vi "AllThingsBaxter_ROS_myRIO.vi"() -> ()   [LabVIEW 2015]
doc: "Collection of all ROS for LabVIEW VIs in the palette"
uses:
  ROS/MessageBuilding/std_msgs/subs/boolScalar.vi
  ROS/MessageBuilding/std_msgs/subs/durationScalar.vi
  ROS/MessageBuilding/std_msgs/subs/float32Scalar.vi
  ROS/MessageBuilding/std_msgs/subs/float64Scalar.vi
  ROS/MessageBuilding/std_msgs/subs/i8Scalar.vi
  ROS/MessageBuilding/std_msgs/subs/i16Scalar.vi
  ROS/MessageBuilding/std_msgs/subs/i32Scalar.vi
  ROS/MessageBuilding/std_msgs/subs/i64Scalar.vi
  ROS/MessageBuilding/std_msgs/subs/stringScalar.vi
  ROS/MessageBuilding/std_msgs/subs/timeScalar.vi
  ROS/MessageBuilding/std_msgs/subs/u8Scalar.vi
  ROS/MessageBuilding/std_msgs/subs/u16Scalar.vi
  ROS/MessageBuilding/std_msgs/subs/u32Scalar.vi
  ROS/MessageBuilding/std_msgs/subs/u64Scalar.vi
  ROS/Code/_ROSDefinition.vi
  ROS/MessageParsing/std_msgs/subs/parse_bool_scalar.vi
  ROS/MessageParsing/std_msgs/subs/parse_duration_scalar.vi
  ROS/MessageParsing/std_msgs/subs/parse_float32_scalar.vi
  ROS/MessageParsing/std_msgs/subs/parse_float64_scalar.vi
  ROS/MessageParsing/std_msgs/subs/parse_i16_scalar.vi
  ROS/MessageParsing/std_msgs/subs/parse_i32_scalar.vi
  ROS/MessageParsing/std_msgs/subs/parse_i64_scalar.vi
  ROS/MessageParsing/std_msgs/subs/parse_i8_scalar.vi
  ROS/MessageParsing/std_msgs/subs/parse_string_scalar.vi
  ROS/MessageParsing/std_msgs/subs/parse_time_scalar.vi
  ROS/MessageParsing/std_msgs/subs/parse_u16_scalar.vi
  ROS/MessageParsing/std_msgs/subs/parse_u32_scalar.vi
  ROS/MessageParsing/std_msgs/subs/parse_u64_scalar.vi
  ROS/MessageParsing/std_msgs/subs/parse_u8_scalar.vi
  ROS/MessageParsing/std_msgs/subs/parse_bool_array.vi
  BaxterVIs/LeftGripper.vi
  BaxterVIs/BothArmsPosition.vi
  BaxterVIs/read_green_level.vi
panel:
  out "ROS Master":string="192.168.1.110:11311"
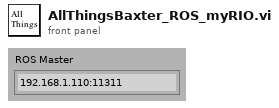
[diagram p1: front panel]
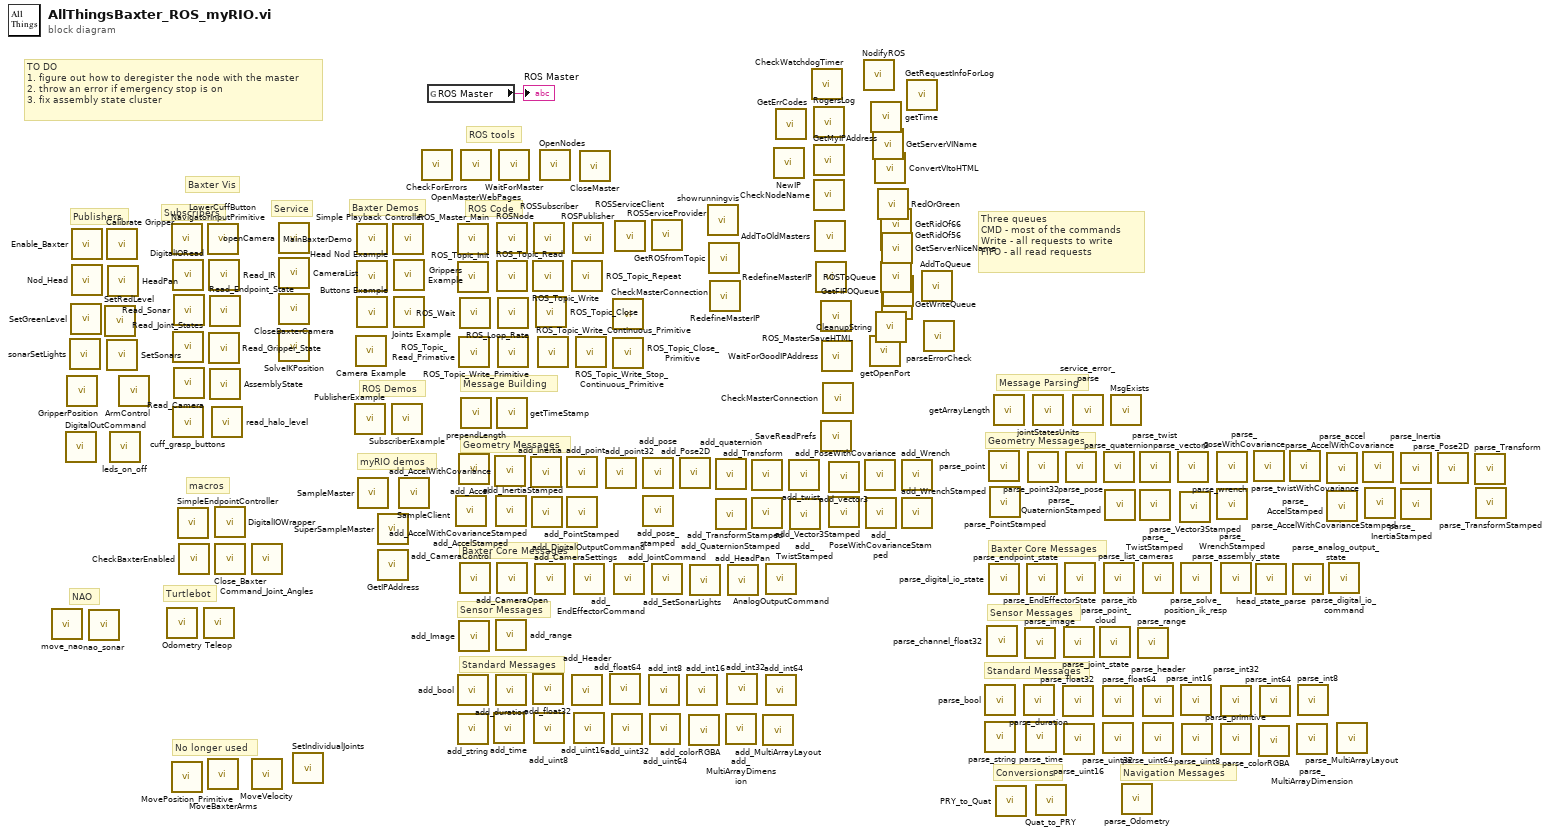
[diagram p0: block diagram]
diagram:
  # "TO DO\n1. figure out how to deregister the node with the master\n2. throw an error if emergency stop is on\n3. fix assembly state cluster"
  # "Navigation Messages"
  # "Turtlebot"
  # "NAO"
  # "No longer used"
  # "Three queues\nCMD - most of the commands\nWrite - all requests to write\nFIFO - all read requests"
  # "Conversions"
  # "Standard Messages"
  # "Sensor Messages"
  # "Geometry Messages"
  # "Baxter Core Messages"
  # "Message Parsing"
  # "myRIO demos"
  # "ROS Demos"
  # "ROS tools"
  # "macros"
  # "Service"
  # "Subscribers"
  # "Publishers"
  # "Standard Messages"
  # "Sensor Messages"
  # "Baxter Core Messages"
  # "Geometry Messages"
  # "Message Building"
  # "ROS Code"
  # "Baxter Demos"
  # "Baxter Vis"
  n1 = call "move_nao.vi"() -> ()  [unwired: 5 in, 1 out]
  n2 = call "DigitalOutCommand.vi"() -> ()  [unwired: 4 in, 1 out]
  n3 = call-poly "GripperPosition.vi"() -> ()  [unwired: 4 in, 1 out]
  n4 = call "sonarSetLights.vi"() -> ()  [unwired: 4 in, 1 out]
  n5 = call "SetGreenLevel.vi"() -> ()  [unwired: 4 in, 1 out]
  n6 = call "Enable_Baxter.vi"() -> ()  [unwired: 4 in, 1 out]
  n7 = call "Nod_Head.vi"() -> ()  [unwired: 4 in, 1 out]
  n8 = call "nao_sonar.vi"() -> ()  [unwired: 4 in, 2 out]
  n9 = call "SetRedLevel.vi"() -> ()  [unwired: 4 in, 1 out]
  n10 = call "Calibrate Gripper.vi"() -> ()  [unwired: 4 in, 1 out]
  n11 = call "SetSonars.vi"() -> ()  [unwired: 4 in, 1 out]
  n12 = call "HeadPan.vi"() -> ()  [unwired: 4 in, 1 out]
  n13 = call "leds_on_off.vi"() -> ()  [unwired: 4 in, 1 out]
  n14 = call-poly "ArmControl.vi"() -> ()  [unwired: 4 in, 1 out]
  n15 = call "Odometry.vi"() -> ()  [unwired: 3 in, 2 out]
  n16 = call "NavigatorInputPrimitive.vi"() -> ()  [unwired: 3 in, 2 out]
  n17 = call "MovePosition_Primitive.vi"() -> ()  [unwired: 6 in, 1 out]
  n18 = call "DigitalIORead.vi"() -> ()  [unwired: 3 in, 2 out]
  n19 = call "Read_Joint_States.vi"() -> ()  [unwired: 3 in, 2 out]
  n20 = call "cuff_grasp_buttons.vi"() -> ()  [unwired: 3 in, 2 out]
  n21 = call "Read_Sonar.vi"() -> ()  [unwired: 3 in, 2 out]
  n22 = call "Read_Camera.vi"() -> ()  [unwired: 4 in, 3 out]
  n23 = call "SimpleEndpointController.vi"() -> ()  [unwired: 5 in, 1 out]
  n24 = call "CheckBaxterEnabled.vi"() -> ()  [unwired: 4 in, 1 out]
  n25 = call "Teleop.vi"() -> ()  [unwired: 4 in, 1 out]
  n26 = call "LowerCuffButton.vi"() -> ()  [unwired: 3 in, 2 out]
  n27 = call "MoveBaxterArms.vi"() -> ()  [unwired: 6 in, 1 out]
  n28 = call "Read_IR.vi"() -> ()  [unwired: 3 in, 2 out]
  n29 = call "Read_Gripper_State.vi"() -> ()  [unwired: 3 in, 2 out]
  n30 = call "Read_Endpoint_State.vi"() -> ()  [unwired: 3 in, 2 out]
  n31 = call "AssemblyState.vi"() -> ()  [unwired: 3 in, 2 out]
  n32 = call-poly "read_halo_level.vi"() -> ()  [unwired: 3 in, 2 out]
  n33 = call "DigitalIOWrapper.vi"() -> ()  [unwired: 3 in, 2 out]
  n34 = call "Close_Baxter.vi"() -> ()  [unwired: 4 in, 1 out]
  n35 = call "Command_Joint_Angles.vi"() -> ()  [unwired: 6 in, 1 out]
  n36 = call "MoveVelocity.vi"() -> ()  [unwired: 6 in, 1 out]
  n37 = call "openCamera.vi"() -> ()  [unwired: 4 in, 1 out]
  n38 = call "CameraList.vi"() -> ()  [unwired: 3 in, 2 out]
  n39 = call "CloseBaxterCamera.vi"() -> ()  [unwired: 4 in, 1 out]
  n40 = call "SolveIKPosition.vi"() -> ()  [unwired: 3 in, 2 out]
  n41 = call "SetIndividualJoints.vi"() -> ()  [unwired: 6 in, 1 out]
  n42 = call "PublisherExample.vi"() -> ()  [unwired: 12 in]
  n43 = call "Camera Example.vi"() -> ()  [unwired: 12 in]
  n44 = call "MainBaxterDemo.vi"() -> ()  [unwired: 12 in]
  n45 = call "Head Nod Example.vi"() -> ()  [unwired: 12 in]
  n46 = call "Buttons Example.vi"() -> ()  [unwired: 12 in]
  n47 = call "SampleMaster.vi"() -> ()  [unwired: 12 in]
  n48 = call "SuperSampleMaster.vi"() -> ()  [unwired: 12 in]
  n49 = call "GetIPAddress.vi"() -> ()  [unwired: 3 in, 1 out]
  n50 = call "SubscriberExample.vi"() -> ()  [unwired: 12 in]
  n51 = call "Simple Playback Controller.vi"() -> ()  [unwired: 12 in]
  n52 = call "Grippers Example.vi"() -> ()  [unwired: 12 in]
  n53 = call "Joints Example.vi"() -> ()  [unwired: 12 in]
  n54 = call "SampleClient.vi"() -> ()  [unwired: 12 in]
  n55 = call "CheckForErrors.vi"() -> ()  [unwired: 2 in, 3 out]
  n56 = global read "_ROSDefinition.vi" "ROS Master"() -> (→"ROS Master":string)
  n57 = call "add_AccelStamped.vi"() -> ()  [unwired: 7 in, 1 out]
  n58 = call "ROS_Master_Main.vi"() -> ()  [unwired: 4 in]
  n59 = call "ROS_Topic_Init.vi"() -> ()  [unwired: 3 in, 2 out]
  n60 = call-poly "add_bool.vi"() -> ()  [unwired: 5 in, 1 out]
  n61 = call-poly "add_string.vi"() -> ()  [unwired: 5 in, 1 out]
  n62 = call "ROS_Topic_Read_Primative.vi"() -> ()  [unwired: 2 in, 3 out]
  n63 = call "add_Accel.vi"() -> ()  [unwired: 7 in, 1 out]
  n64 = call "add_Image.vi"() -> ()  [unwired: 5 in, 1 out]
  n65 = call "ROS_Wait.vi"() -> ()  [unwired: 3 in, 2 out]
  n66 = call "add_CameraControl.vi"() -> ()  [unwired: 5 in, 1 out]
  n67 = call "OpenMasterWebPages.vi"() -> ()  [unwired: 4 in]
  n68 = call "prependLength.vi"() -> ()  [unwired: 5 in, 1 out]
  n69 = call-poly "add_time.vi"() -> ()  [unwired: 5 in, 1 out]
  n70 = call "add_AccelWithCovariance.vi"() -> ()  [unwired: 7 in, 1 out]
  n71 = call "add_AccelWithCovarianceStamped.vi"() -> ()  [unwired: 7 in, 1 out]
  n72 = call "add_range.vi"() -> ()  [unwired: 7 in, 1 out]
  n73 = call-poly "add_duration.vi"() -> ()  [unwired: 5 in, 1 out]
  n74 = call "ROSNode.vi"() -> ()  [unwired: 4 in]
  n75 = call "ROS_Topic_Read.vi"() -> ()  [unwired: 3 in, 3 out]
  n76 = call "getTimeStamp.vi"() -> ()  [unwired: 2 in, 3 out]
  n77 = call "add_CameraOpen.vi"() -> ()  [unwired: 5 in, 1 out]
  n78 = call "ROS_Loop_Rate.vi"() -> ()  [unwired: 5 in, 2 out]
  n79 = call "ROS_Topic_Write_Primitive.vi"() -> ()  [unwired: 3 in, 1 out]
  n80 = call "WaitForMaster.vi"() -> ()  [unwired: 1 in, 1 out]
  n81 = call "add_Inertia.vi"() -> ()  [unwired: 7 in, 1 out]
  n82 = call "add_InertiaStamped.vi"() -> ()  [unwired: 7 in, 1 out]
  n83 = call "ROS_Topic_Write.vi"() -> ()  [unwired: 4 in, 2 out]
  n84 = call-poly "add_float32.vi"() -> ()  [unwired: 5 in, 1 out]
  n85 = call "ROSSubscriber.vi"() -> ()  [unwired: 4 in]
  n86 = call-poly "add_uint8.vi"() -> ()  [unwired: 5 in, 1 out]
  n87 = call "add_CameraSettings.vi"() -> ()  [unwired: 5 in, 1 out]
  n88 = call "ROS_Topic_Close.vi"() -> ()  [unwired: 4 in, 1 out]
  n89 = call "ROS_Topic_Write_Continuous_Primitive.vi"() -> ()  [unwired: 3 in, 1 out]
  n90 = call "OpenNodes.vi"() -> ()  [unwired: 2 in]
  n91 = call "add_point.vi"() -> ()  [unwired: 5 in, 1 out]
  n92 = call "add_PointStamped.vi"() -> ()  [unwired: 7 in, 1 out]
  n93 = call "ROS_Topic_Repeat.vi"() -> ()  [unwired: 4 in, 2 out]
  n94 = call "add_Header.vi"() -> ()  [unwired: 5 in, 1 out]
  n95 = call "ROSPublisher.vi"() -> ()  [unwired: 4 in]
  n96 = call "add_DigitalOutputCommand.vi"() -> ()  [unwired: 5 in, 1 out]
  n97 = call-poly "add_uint16.vi"() -> ()  [unwired: 5 in, 1 out]
  n98 = call "ROS_Topic_Write_Stop_Continuous_Primitive.vi"() -> ()  [unwired: 3 in, 1 out]
  n99 = call "CloseMaster.vi"() -> ()  [unwired: 3 in, 1 out]
  n100 = call "add_point32.vi"() -> ()  [unwired: 7 in, 1 out]
  n101 = call-poly "add_float64.vi"() -> ()  [unwired: 5 in, 1 out]
  n102 = call-poly "add_uint32.vi"() -> ()  [unwired: 5 in, 1 out]
  n103 = call "CheckMasterConnection.vi"() -> ()  [unwired: 2 in, 2 out]
  n104 = call "ROS_Topic_Close_Primitive.vi"() -> ()  [unwired: 3 in, 1 out]
  n105 = call "add_EndEffectorCommand.vi"() -> ()  [unwired: 5 in, 1 out]
  n106 = call "ROSServiceClient.vi"() -> ()  [unwired: 4 in]
  n107 = call "add_pose.vi"() -> ()  [unwired: 5 in, 1 out]
  n108 = call "add_pose_stamped.vi"() -> ()  [unwired: 5 in, 1 out]
  n109 = call-poly "add_int8.vi"() -> ()  [unwired: 5 in, 1 out]
  n110 = call-poly "add_uint64.vi"() -> ()  [unwired: 5 in, 1 out]
  n111 = call "ROSServiceProvider.vi"() -> ()  [unwired: 4 in]
  n112 = call "add_JointCommand.vi"() -> ()  [unwired: 11 in, 1 out]
  n113 = call "add_Pose2D.vi"() -> ()  [unwired: 7 in, 1 out]
  n114 = call-poly "add_int16.vi"() -> ()  [unwired: 5 in, 1 out]
  n115 = call "add_colorRGBA.vi"() -> ()  [unwired: 7 in, 1 out]
  n116 = call "add_SetSonarLights.vi"() -> ()  [unwired: 5 in, 1 out]
  n117 = call "showrunningvis.vi"() -> ()  [unwired: 1 in]
  n118 = call "GetROSfromTopic.vi"() -> ()  [unwired: 2 in, 3 out]
  n119 = call "RedefineMasterIP.vi"() -> ()  [unwired: 2 in, 1 out]
  n120 = call "add_quaternion.vi"() -> ()  [unwired: 5 in, 1 out]
  n121 = call "add_QuaternionStamped.vi"() -> ()  [unwired: 7 in, 1 out]
  n122 = call "add_MultiArrayDimension.vi"() -> ()  [unwired: 7 in, 1 out]
  n123 = call-poly "add_int32.vi"() -> ()  [unwired: 5 in, 1 out]
  n124 = call "add_HeadPan.vi"() -> ()  [unwired: 11 in, 1 out]
  n125 = call "add_Transform.vi"() -> ()  [unwired: 7 in, 1 out]
  n126 = call "add_TransformStamped.vi"() -> ()  [unwired: 7 in, 1 out]
  n127 = call "add_MultiArrayLayout.vi"() -> ()  [unwired: 7 in, 1 out]
  n128 = call "AnalogOutputCommand.vi"() -> ()  [unwired: 7 in, 1 out]
  n129 = call-poly "add_int64.vi"() -> ()  [unwired: 5 in, 1 out]
  n130 = call "NewIP.vi"() -> ()  [unwired: 2 in, 2 out]
  n131 = call "GetErrCodes.vi"() -> ()  [unwired: 2 in, 1 out]
  n132 = call "add_twist.vi"() -> ()  [unwired: 5 in, 1 out]
  n133 = call "add_TwistStamped.vi"() -> ()  [unwired: 7 in, 1 out]
  n134 = call "CheckWatchdogTimer.vi"() -> ()  [unwired: 6 in]
  n135 = call "RogersLog.vi"() -> ()  [unwired: 5 in, 2 out]
  n136 = call "GetMyIPAddress.vi"() -> ()  [unwired: 2 in, 2 out]
  n137 = call "CheckNodeName.vi"() -> ()  [unwired: 2 in, 2 out]
  n138 = call "AddToOldMasters.vi"() -> ()  [unwired: 4 in]
  n139 = call "RedefineMasterIP.vi"() -> ()  [unwired: 2 in, 1 out]
  n140 = call "ROS_MasterSaveHTML.vi"() -> ()  [unwired: 6 in]
  n141 = call "SaveReadPrefs.vi"() -> ()  [unwired: 3 in, 1 out]
  n142 = call "WaitForGoodIPAddress.vi"() -> ()  [unwired: 1 in, 1 out]
  n143 = call "CheckMasterConnection.vi"() -> ()  [unwired: 2 in, 2 out]
  n144 = call "add_vector3.vi"() -> ()  [unwired: 5 in, 1 out]
  n145 = call "add_Vector3Stamped.vi"() -> ()  [unwired: 7 in, 1 out]
  n146 = call "NodifyROS.vi"() -> ()  [unwired: 1 in, 1 out]
  n147 = call "add_PoseWithCovariance.vi"() -> ()  [unwired: 5 in, 1 out]
  n148 = call "add_PoseWithCovarianceStamped.vi"() -> ()  [unwired: 7 in, 1 out]
  n149 = call "getOpenPort.vi"() -> ()  [unwired: 1 out]
  n150 = call "getTime.vi"() -> ()  [unwired: 1 in, 1 out]
  n151 = call "GetServerVIName.vi"() -> ()  [unwired: 1 in, 1 out]
  n152 = call "ConvertVItoHTML.vi"() -> ()  [unwired: 1 in, 2 out]
  n153 = call "CleanupString.vi"() -> ()  [unwired: 1 in, 1 out]
  n154 = call "RedOrGreen.vi"() -> ()  [unwired: 1 in, 1 out]
  n155 = call "GetRidOf66.vi"() -> ()  [unwired: 1 in, 1 out]
  n156 = call "GetRidOf56.vi"() -> ()  [unwired: 1 in, 1 out]
  n157 = call "ROSToQueue.vi"() -> ()  [unwired: 4 in, 2 out]
  n158 = call "GetServerNiceName.vi"() -> ()  [unwired: 2 in, 1 out]
  n159 = call "GetWriteQueue.vi"() -> ()  [unwired: 4 in, 2 out]
  n160 = call "GetFIFOQueue.vi"() -> ()  [unwired: 4 in, 2 out]
  n161 = call "add_Wrench.vi"() -> ()  [unwired: 5 in, 1 out]
  n162 = call "add_WrenchStamped.vi"() -> ()  [unwired: 7 in, 1 out]
  n163 = call "GetRequestInfoForLog.vi"() -> ()  [unwired: 1 in, 1 out]
  n164 = call "AddToQueue.vi"() -> ()  [unwired: 5 in, 1 out]
  n165 = call "parseErrorCheck.vi"() -> ()  [unwired: 3 in, 1 out]
  n166 = call-poly "parse_bool.vi"() -> ()  [unwired: 5 in, 3 out]
  n167 = call-poly "parse_string.vi"() -> ()  [unwired: 5 in, 3 out]
  n168 = call "parse_channel_float32.vi"() -> ()  [unwired: 5 in, 3 out]
  n169 = call "parse_point.vi"() -> ()  [unwired: 5 in, 3 out]
  n170 = call "parse_digital_io_state.vi"() -> ()  [unwired: 5 in, 3 out]
  n171 = call "parse_PointStamped.vi"() -> ()  [unwired: 5 in, 3 out]
  n172 = call "getArrayLength.vi"() -> ()  [unwired: 5 in, 3 out]
  n173 = call "PRY_to_Quat.vi"() -> ()  [unwired: 2 in, 1 out]
  n174 = call-poly "parse_duration.vi"() -> ()  [unwired: 5 in, 3 out]
  n175 = call "parse_image.vi"() -> ()  [unwired: 4 in, 4 out]
  n176 = call-poly "parse_time.vi"() -> ()  [unwired: 5 in, 3 out]
  n177 = call "parse_endpoint_state.vi"() -> ()  [unwired: 5 in, 3 out]
  n178 = call "parse_point32.vi"() -> ()  [unwired: 5 in, 3 out]
  n179 = call "jointStatesUnits.vi"() -> ()  [unwired: 3 in, 3 out]
  n180 = call "Quat_to_PRY.vi"() -> ()  [unwired: 2 in, 1 out]
  n181 = call-poly "parse_float32.vi"() -> ()  [unwired: 5 in, 3 out]
  n182 = call "parse_joint_state.vi"() -> ()  [unwired: 4 in, 4 out]
  n183 = call-poly "parse_uint16.vi"() -> ()  [unwired: 5 in, 3 out]
  n184 = call "parse_EndEffectorState.vi"() -> ()  [unwired: 5 in, 3 out]
  n185 = call "parse_pose.vi"() -> ()  [unwired: 5 in, 3 out]
  n186 = call "service_error_parse.vi"() -> ()  [unwired: 3 in, 3 out]
  n187 = call "parse_point_cloud.vi"() -> ()  [unwired: 4 in, 4 out]
  n188 = call-poly "parse_float64.vi"() -> ()  [unwired: 5 in, 3 out]
  n189 = call-poly "parse_uint32.vi"() -> ()  [unwired: 5 in, 3 out]
  n190 = call "parse_quaternion.vi"() -> ()  [unwired: 5 in, 3 out]
  n191 = call "parse_itb.vi"() -> ()  [unwired: 5 in, 3 out]
  n192 = call "parse_QuaternionStamped.vi"() -> ()  [unwired: 5 in, 3 out]
  n193 = call "MsgExists.vi"() -> ()  [unwired: 10 in, 2 out]
  n194 = call "parse_Odometry.vi"() -> ()  [unwired: 5 in, 5 out]
  n195 = call "parse_range.vi"() -> ()  [unwired: 4 in, 4 out]
  n196 = call "parse_twist.vi"() -> ()  [unwired: 5 in, 3 out]
  n197 = call "parse_TwistStamped.vi"() -> ()  [unwired: 4 in, 4 out]
  n198 = call "parse_list_cameras.vi"() -> ()  [unwired: 5 in, 3 out]
  n199 = call "parse_header.vi"() -> ()  [unwired: 5 in, 3 out]
  n200 = call-poly "parse_uint64.vi"() -> ()  [unwired: 5 in, 3 out]
  n201 = call "parse_vector3.vi"() -> ()  [unwired: 5 in, 3 out]
  n202 = call "parse_Vector3Stamped.vi"() -> ()  [unwired: 4 in, 4 out]
  n203 = call "parse_solve_position_ik_resp.vi"() -> ()  [unwired: 4 in, 4 out]
  n204 = call-poly "parse_int16.vi"() -> ()  [unwired: 5 in, 3 out]
  n205 = call-poly "parse_uint8.vi"() -> ()  [unwired: 5 in, 3 out]
  n206 = call "parse_wrench.vi"() -> ()  [unwired: 5 in, 3 out]
  n207 = call "parse_WrenchStamped.vi"() -> ()  [unwired: 4 in, 4 out]
  n208 = call "parse_assembly_state.vi"() -> ()  [unwired: 4 in, 3 out]
  n209 = call-poly "parse_int32.vi"() -> ()  [unwired: 5 in, 3 out]
  n210 = call-poly "parse_primitive.vi"() -> ()  [unwired: 5 in, 3 out]
  n211 = call "parse_poseWithCovariance.vi"() -> ()  [unwired: 5 in, 3 out]
  n212 = call "head_state_parse.vi"() -> ()  [unwired: 4 in, 4 out]
  n213 = call "parse_colorRGBA.vi"() -> ()  [unwired: 5 in, 3 out]
  n214 = call-poly "parse_int64.vi"() -> ()  [unwired: 5 in, 3 out]
  n215 = call "parse_twistWithCovariance.vi"() -> ()  [unwired: 5 in, 3 out]
  n216 = call "parse_analog_output_state.vi"() -> ()  [unwired: 5 in, 3 out]
  n217 = call "parse_MultiArrayDimension.vi"() -> ()  [unwired: 5 in, 3 out]
  n218 = call-poly "parse_int8.vi"() -> ()  [unwired: 5 in, 3 out]
  n219 = call "parse_accel.vi"() -> ()  [unwired: 5 in, 3 out]
  n220 = call "parse_AccelStamped.vi"() -> ()  [unwired: 4 in, 4 out]
  n221 = call "parse_digital_io_command.vi"() -> ()  [unwired: 5 in, 3 out]
  n222 = call "parse_MultiArrayLayout.vi"() -> ()  [unwired: 4 in, 4 out]
  n223 = call "parse_AccelWithCovariance.vi"() -> ()  [unwired: 5 in, 3 out]
  n224 = call "parse_AccelWithCovarianceStamped.vi"() -> ()  [unwired: 4 in, 4 out]
  n225 = call "parse_Inertia.vi"() -> ()  [unwired: 5 in, 3 out]
  n226 = call "parse_InertiaStamped.vi"() -> ()  [unwired: 4 in, 4 out]
  n227 = call "parse_Pose2D.vi"() -> ()  [unwired: 5 in, 3 out]
  n228 = call "parse_Transform.vi"() -> ()  [unwired: 5 in, 3 out]
  n229 = call "parse_TransformStamped.vi"() -> ()  [unwired: 5 in, 5 out]
